vi "Update Background.vi"(10 "Numeric 2":u16, 11 "Application in":refnum<class "Application.lvclass">) -> ()   [LabVIEW 2021]
uses:
  Application.lvclass
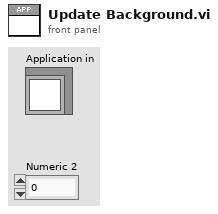
[diagram p1: front panel]
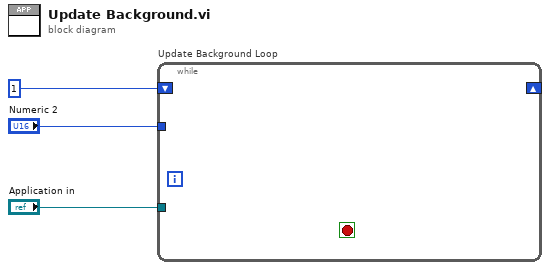
[diagram p0: block diagram]
diagram:
  n1 = while "Update Background Loop" {
    tunnel: "Application in" -> [_]
    shift-right: _ -> [_]
    shift-left: 1 ("Numeric") -> [_]
    tunnel: "Numeric 2" -> [_]
    stop <- _ stop-if-true
  }
